vi "user initialization.vi"(8 "error in":errorcluster, 10 "configuration in":refnum<class "control module configuration.lvclass">, 11 "fixed channel runtime in":refnum<class "CentralErrorHandler runtime.lvclass">) -> (0 "error out":errorcluster, 3 "fixed channel runtime out":refnum<class "CentralErrorHandler runtime.lvclass">)   [LabVIEW 2017, in "CentralErrorHandler runtime.lvclass"]
uses:
  CentralErrorHandler runtime.lvclass
  <vilib>/NI/DCAF/Tag Editor Core/control module/configuration/control module configuration.lvclass
  <vilib>/NI/DCAF/Tag Editor Core/control module/runtime/control module runtime.lvclass
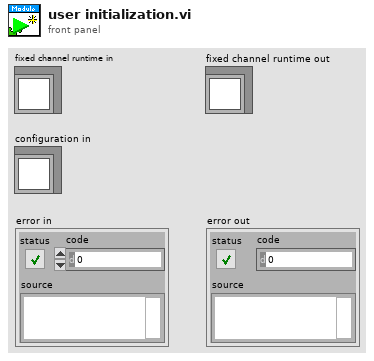
[diagram p1: front panel]
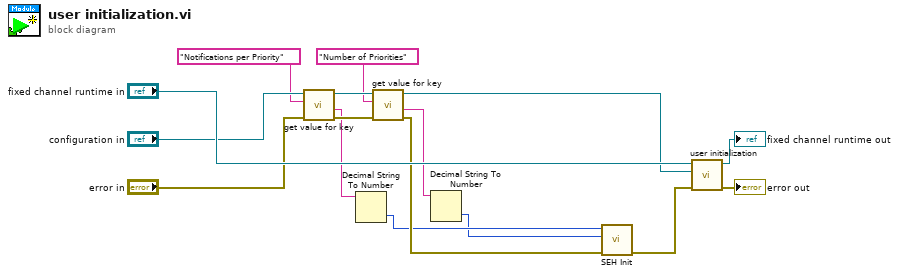
[diagram p0: block diagram]
diagram:
  n1 = call-dynamic "get value for key.vi"("error in"="error in", "key"="Notifications per Priority", "fixed channel configuration in"="configuration in") -> ("error out"=w13:errorcluster, "value"=w4:string, "fixed channel configuration out"=w10:refnum<class "control module configuration.lvclass">)  [unwired: 6 in]
  n2 = Decimal String To Number(string=w4) -> (number=w2:i32)  [unwired: 2 in, 1 out]
  n3 = call-dynamic "get value for key.vi"("error in"=w13, "key"="Number of Priorities", "fixed channel configuration in"=w10) -> ("error out"=w6:errorcluster, "value"=w3:string, "fixed channel configuration out"=w9:refnum<class "control module configuration.lvclass">)  [unwired: 6 in]
  n4 = Decimal String To Number(string=w3) -> (number=w1:i32)  [unwired: 2 in, 1 out]
  n5 = call <userlib>:"SEH Init.vi"("error in (no error)"=w6, "Number of Priorities"=w1, "Notifications per Priority"=w2) -> ("error out"=w5:errorcluster)  [unwired: 8 in]
  n6 = call-parent "user initialization.vi"("error in"=w5, "configuration in"=w9, "fixed channel runtime in"="fixed channel runtime in") -> ("error out"=→"error out":errorcluster, "fixed channel runtime out"=→"fixed channel runtime out":refnum<class "CentralErrorHandler runtime.lvclass">)  [unwired: 7 in]
